vi "外观.vi"(0 "Data In":T9 caption="数据输入", 2 "Display State In":T2 caption="显示状态输入" {"配置信息"."间隔启动"."启动命令" items=["", "水样测试", "标样核查", "零点核查", "跨度核查", "空白测试", "平行样测试", "加标回收", "空白校准", "标样校准"]; "配置信息"."定点周期"."启动命令 24" items=["", "水样测试", "标样核查", "零点核查", "跨度核查", "空白测试", "平行样测试", "加标回收", "空白校准", "标样校准"]; "配置信息"."定点周期"."启动命令 23" items=["", "水样测试", "标样核查", "零点核查", "跨度核查", "空白测试", "平行样测试", "加标回收", "空白校准", "标样校准"]; "配置信息"."定点周期"."启动命令 22" items=["", "水样测试", "标样核查", "零点核查", "跨度核查", "空白测试", "平行样测试", "加标回收", "空白校准", "标样校准"]; "配置信息"."定点周期"."启动命令 21" items=["", "水样测试", "标样核查", "零点核查", "跨度核查", "空白测试", "平行样测试", "加标回收", "空白校准", "标样校准"]; "配置信息"."定点周期"."启动命令 20" items=["", "水样测试", "标样核查", "零点核查", "跨度核查", "空白测试", "平行样测试", "加标回收", "空白校准", "标样校准"]; "配置信息"."定点周期"."启动命令 19" items=["", "水样测试", "标样核查", "零点核查", "跨度核查", "空白测试", "平行样测试", "加标回收", "空白校准", "标样校准"]; "配置信息"."定点周期"."启动命令 18" items=["", "水样测试", "标样核查", "零点核查", "跨度核查", "空白测试", "平行样测试", "加标回收", "空白校准", "标样校准"]; "配置信息"."定点周期"."启动命令 17" items=["", "水样测试", "标样核查", "零点核查", "跨度核查", "空白测试", "平行样测试", "加标回收", "空白校准", "标样校准"]; "配置信息"."定点周期"."启动命令 16" items=["", "水样测试", "标样核查", "零点核查", "跨度核查", "空白测试", "平行样测试", "加标回收", "空白校准", "标样校准"]; "配置信息"."定点周期"."启动命令 15" items=["", "水样测试", "标样核查", "零点核查", "跨度核查", "空白测试", "平行样测试", "加标回收", "空白校准", "标样校准"]; "配置信息"."定点周期"."启动命令 14" items=["", "水样测试", "标样核查", "零点核查", "跨度核查", "空白测试", "平行样测试", "加标回收", "空白校准", "标样校准"]; "配置信息"."定点周期"."启动命令 13" items=["", "水样测试", "标样核查", "零点核查", "跨度核查", "空白测试", "平行样测试", "加标回收", "空白校准", "标样校准"]; "配置信息"."定点周期"."启动命令 12" items=["", "水样测试", "标样核查", "零点核查", "跨度核查", "空白测试", "平行样测试", "加标回收", "空白校准", "标样校准"]; "配置信息"."定点周期"."启动命令 11" items=["", "水样测试", "标样核查", "零点核查", "跨度核查", "空白测试", "平行样测试", "加标回收", "空白校准", "标样校准"]; "配置信息"."定点周期"."启动命令 10" items=["", "水样测试", "标样核查", "零点核查", "跨度核查", "空白测试", "平行样测试", "加标回收", "空白校准", "标样校准"]; "配置信息"."定点周期"."启动命令 9" items=["", "水样测试", "标样核查", "零点核查", "跨度核查", "空白测试", "平行样测试", "加标回收", "空白校准", "标样校准"]; "配置信息"."定点周期"."启动命令 8" items=["", "水样测试", "标样核查", "零点核查", "跨度核查", "空白测试", "平行样测试", "加标回收", "空白校准", "标样校准"]; "配置信息"."定点周期"."启动命令 7" items=["", "水样测试", "标样核查", "零点核查", "跨度核查", "空白测试", "平行样测试", "加标回收", "空白校准", "标样校准"]; "配置信息"."定点周期"."启动命令 6" items=["", "水样测试", "标样核查", "零点核查", "跨度核查", "空白测试", "平行样测试", "加标回收", "空白校准", "标样校准"]; "配置信息"."定点周期"."启动命令 5" items=["", "水样测试", "标样核查", "零点核查", "跨度核查", "空白测试", "平行样测试", "加标回收", "空白校准", "标样校准"]; "配置信息"."定点周期"."启动命令 4" items=["", "水样测试", "标样核查", "零点核查", "跨度核查", "空白测试", "平行样测试", "加标回收", "空白校准", "标样校准"]; "配置信息"."定点周期"."启动命令 3" items=["", "水样测试", "标样核查", "零点核查", "跨度核查", "空白测试", "平行样测试", "加标回收", "空白校准", "标样校准"]; "配置信息"."定点周期"."启动命令 2" items=["", "水样测试", "标样核查", "零点核查", "跨度核查", "空白测试", "平行样测试", "加标回收", "空白校准", "标样校准"]; "配置信息"."定点周期"."启动命令" items=["", "水样测试", "标样核查", "零点核查", "跨度核查", "空白测试", "平行样测试", "加标回收", "空白校准", "标样校准"]}, 3 "Container State":T8 caption="容器状态") -> (6 "Data Out":T9 caption="数据输出", 7 "Display State Out":T2 caption="显示状态输出" {"配置信息"."间隔启动"."启动命令" items=["", "水样测试", "标样核查", "零点核查", "跨度核查", "空白测试", "平行样测试", "加标回收", "空白校准", "标样校准"]; "配置信息"."定点周期"."启动命令 24" items=["", "水样测试", "标样核查", "零点核查", "跨度核查", "空白测试", "平行样测试", "加标回收", "空白校准", "标样校准"]; "配置信息"."定点周期"."启动命令 23" items=["", "水样测试", "标样核查", "零点核查", "跨度核查", "空白测试", "平行样测试", "加标回收", "空白校准", "标样校准"]; "配置信息"."定点周期"."启动命令 22" items=["", "水样测试", "标样核查", "零点核查", "跨度核查", "空白测试", "平行样测试", "加标回收", "空白校准", "标样校准"]; "配置信息"."定点周期"."启动命令 21" items=["", "水样测试", "标样核查", "零点核查", "跨度核查", "空白测试", "平行样测试", "加标回收", "空白校准", "标样校准"]; "配置信息"."定点周期"."启动命令 20" items=["", "水样测试", "标样核查", "零点核查", "跨度核查", "空白测试", "平行样测试", "加标回收", "空白校准", "标样校准"]; "配置信息"."定点周期"."启动命令 19" items=["", "水样测试", "标样核查", "零点核查", "跨度核查", "空白测试", "平行样测试", "加标回收", "空白校准", "标样校准"]; "配置信息"."定点周期"."启动命令 18" items=["", "水样测试", "标样核查", "零点核查", "跨度核查", "空白测试", "平行样测试", "加标回收", "空白校准", "标样校准"]; "配置信息"."定点周期"."启动命令 17" items=["", "水样测试", "标样核查", "零点核查", "跨度核查", "空白测试", "平行样测试", "加标回收", "空白校准", "标样校准"]; "配置信息"."定点周期"."启动命令 16" items=["", "水样测试", "标样核查", "零点核查", "跨度核查", "空白测试", "平行样测试", "加标回收", "空白校准", "标样校准"]; "配置信息"."定点周期"."启动命令 15" items=["", "水样测试", "标样核查", "零点核查", "跨度核查", "空白测试", "平行样测试", "加标回收", "空白校准", "标样校准"]; "配置信息"."定点周期"."启动命令 14" items=["", "水样测试", "标样核查", "零点核查", "跨度核查", "空白测试", "平行样测试", "加标回收", "空白校准", "标样校准"]; "配置信息"."定点周期"."启动命令 13" items=["", "水样测试", "标样核查", "零点核查", "跨度核查", "空白测试", "平行样测试", "加标回收", "空白校准", "标样校准"]; "配置信息"."定点周期"."启动命令 12" items=["", "水样测试", "标样核查", "零点核查", "跨度核查", "空白测试", "平行样测试", "加标回收", "空白校准", "标样校准"]; "配置信息"."定点周期"."启动命令 11" items=["", "水样测试", "标样核查", "零点核查", "跨度核查", "空白测试", "平行样测试", "加标回收", "空白校准", "标样校准"]; "配置信息"."定点周期"."启动命令 10" items=["", "水样测试", "标样核查", "零点核查", "跨度核查", "空白测试", "平行样测试", "加标回收", "空白校准", "标样校准"]; "配置信息"."定点周期"."启动命令 9" items=["", "水样测试", "标样核查", "零点核查", "跨度核查", "空白测试", "平行样测试", "加标回收", "空白校准", "标样校准"]; "配置信息"."定点周期"."启动命令 8" items=["", "水样测试", "标样核查", "零点核查", "跨度核查", "空白测试", "平行样测试", "加标回收", "空白校准", "标样校准"]; "配置信息"."定点周期"."启动命令 7" items=["", "水样测试", "标样核查", "零点核查", "跨度核查", "空白测试", "平行样测试", "加标回收", "空白校准", "标样校准"]; "配置信息"."定点周期"."启动命令 6" items=["", "水样测试", "标样核查", "零点核查", "跨度核查", "空白测试", "平行样测试", "加标回收", "空白校准", "标样校准"]; "配置信息"."定点周期"."启动命令 5" items=["", "水样测试", "标样核查", "零点核查", "跨度核查", "空白测试", "平行样测试", "加标回收", "空白校准", "标样校准"]; "配置信息"."定点周期"."启动命令 4" items=["", "水样测试", "标样核查", "零点核查", "跨度核查", "空白测试", "平行样测试", "加标回收", "空白校准", "标样校准"]; "配置信息"."定点周期"."启动命令 3" items=["", "水样测试", "标样核查", "零点核查", "跨度核查", "空白测试", "平行样测试", "加标回收", "空白校准", "标样校准"]; "配置信息"."定点周期"."启动命令 2" items=["", "水样测试", "标样核查", "零点核查", "跨度核查", "空白测试", "平行样测试", "加标回收", "空白校准", "标样校准"]; "配置信息"."定点周期"."启动命令" items=["", "水样测试", "标样核查", "零点核查", "跨度核查", "空白测试", "平行样测试", "加标回收", "空白校准", "标样校准"]}, 8 "Action":T1 caption="动作")   [LabVIEW 2016, in "定时设置.xctl"]
uses:
  <vilib>/_xctls/Container State.ctl
  <vilib>/_xctls/Action.ctl
  <vilib>/Utility/miscctls.llb/LVPositionTypeDef.ctl
  <vilib>/_xctls/XControlSupport.lvlib
  <vilib>/ptbypt/NI_PtbyPt.lvlib
panel:
  in  "周期设置":bool
  # "分钟"
  # "次"
  # "分钟"
  # "次"
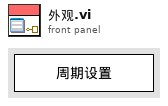
[diagram p1: front panel]
types:
  T1 = typedef "XControlSupport.lvlib/Action.ctl" = cluster{"Data Changed?":bool, "State Changed?":bool, "Action Name":string}
  T2 = typedef "定时设置.xctl/状态.ctl" = cluster{"配置信息":cluster{"周期模式":T3, "定点周期":T4, "间隔启动":T6, "测量参数":T7}, "仪器运行状态":bool, "启动次数":i32, "最近一次启动时间":timestamp, "最近一次结束时间":timestamp, "间隔计时":dbl, "测量参数名称":string[], "时间源":cluster{"时间源选择":enum16{"系统时间源", "仪器时间源"}, "外部时间源":timestamp}, "引用参数":string}
  T3 = typedef "定时设置.xctl/周期模式设置.ctl" = enum16{"不启用", "定点模式", "间隔模式"}
  T4 = typedef "定时设置.xctl/定点周期设置.ctl" = cluster{"启动命令":T5, "启动命令 2":T5, "启动命令 3":T5, "启动命令 4":T5, "启动命令 5":T5, "启动命令 6":T5, "启动命令 7":T5, "启动命令 8":T5, "启动命令 9":T5, "启动命令 10":T5, "启动命令 11":T5, "启动命令 12":T5, "启动命令 13":T5, "启动命令 14":T5, "启动命令 15":T5, "启动命令 16":T5, "启动命令 17":T5, "启动命令 18":T5, "启动命令 19":T5, "启动命令 20":T5, "启动命令 21":T5, "启动命令 22":T5, "启动命令 23":T5, "启动命令 24":T5}
  T5 = typedef "定时设置.xctl/启动命令选择.ctl" = u16
  T6 = typedef "定时设置.xctl/间隔启动设置.ctl" = cluster{"启动命令":T5, "启动间隔":dbl, "启动次数":i32}
  T7 = typedef "定时设置.xctl/测量参数.ctl" = u16
  T8 = typedef "XControlSupport.lvlib/Container State.ctl" = cluster{"Indicator?":bool, "Run Mode?":bool, " Refnum":refnum<vi>}
  T9 = typedef "定时设置.xctl/数据.ctl" = cluster{"启动":bool, "控制命令":T10, "测量参数":T7}
  T10 = typedef "定时设置.xctl/国标控制命令.ctl" = enum16{"启动测量", "标样核查", "零点核查", "跨度核查", "空白测试", "平行样测试", "加标回收", "空白校准", "标样校准", "初始化（清洗）", "停止测试", "仪器重启", "校时", "模式设置", "测量间隔设置"}
  T11 = typedef "LVPositionTypeDef.ctl" = cluster{"Left":i32, "Top":i32}
  T12 = cluster{"周期模式":T3, "定点周期":T4, "间隔设置":cluster{"启动命令":T5, "启动间隔":dbl, "启动次数":i32}, "测量参数":T7}
  T13 = cluster{"周期模式":T3, "定点周期":T4, "间隔启动":T6, "测量参数":T7}
  T14 = cluster{"时间源选择":enum16{"系统时间源", "仪器时间源"}, "外部时间源":timestamp}
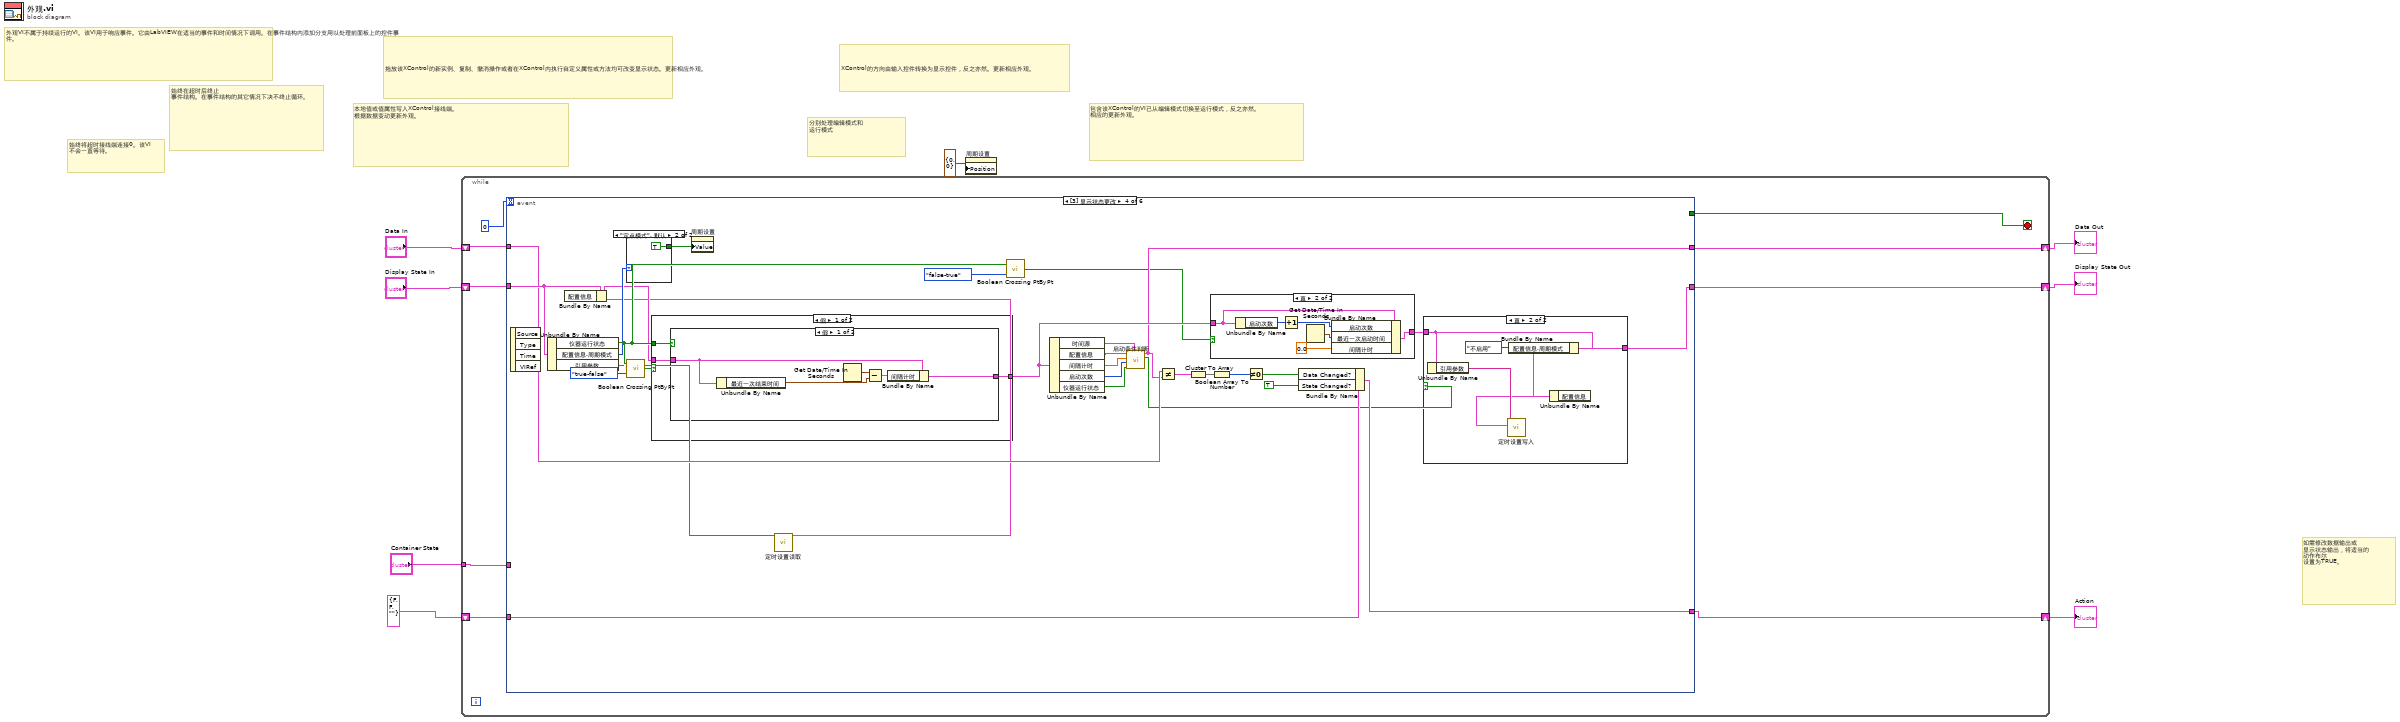
[diagram p0: block diagram]
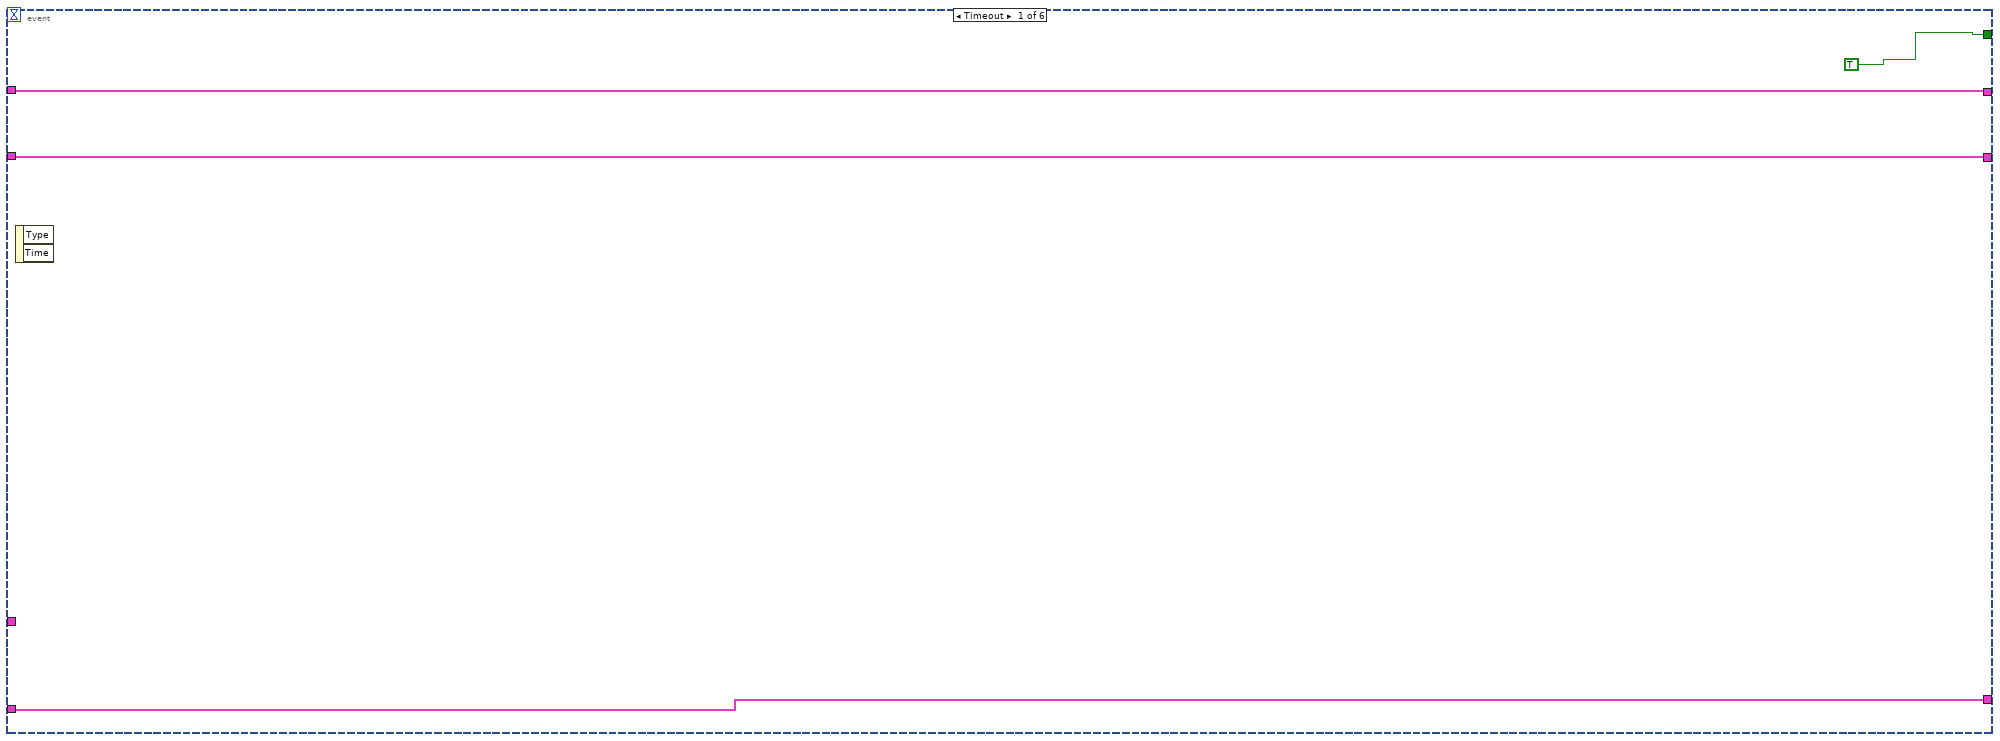
[diagram p2: hidden frame]
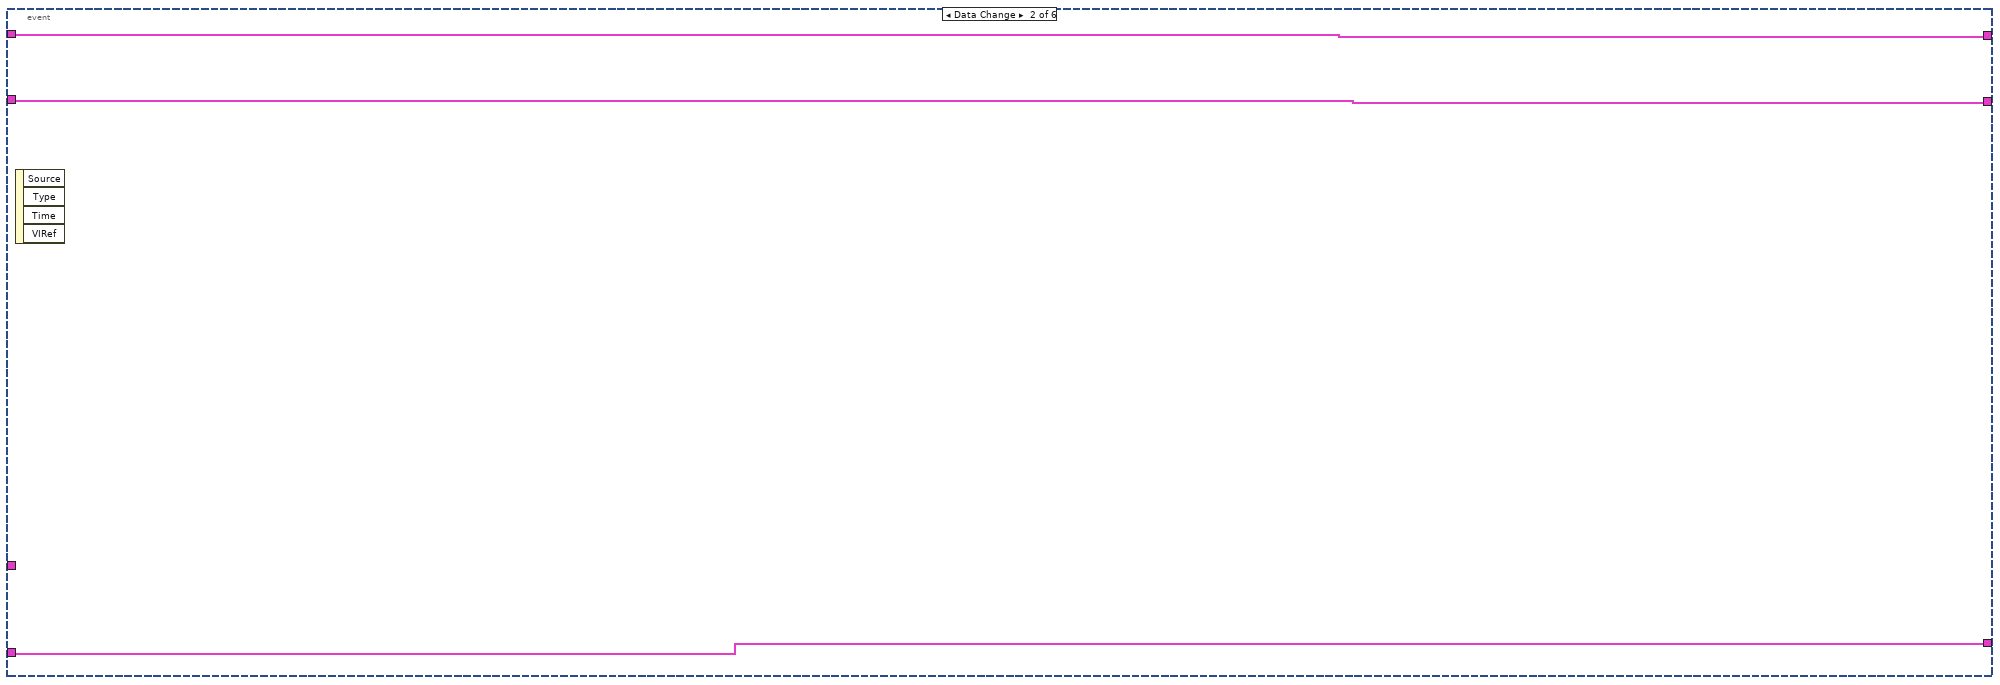
[diagram p3: hidden frame]
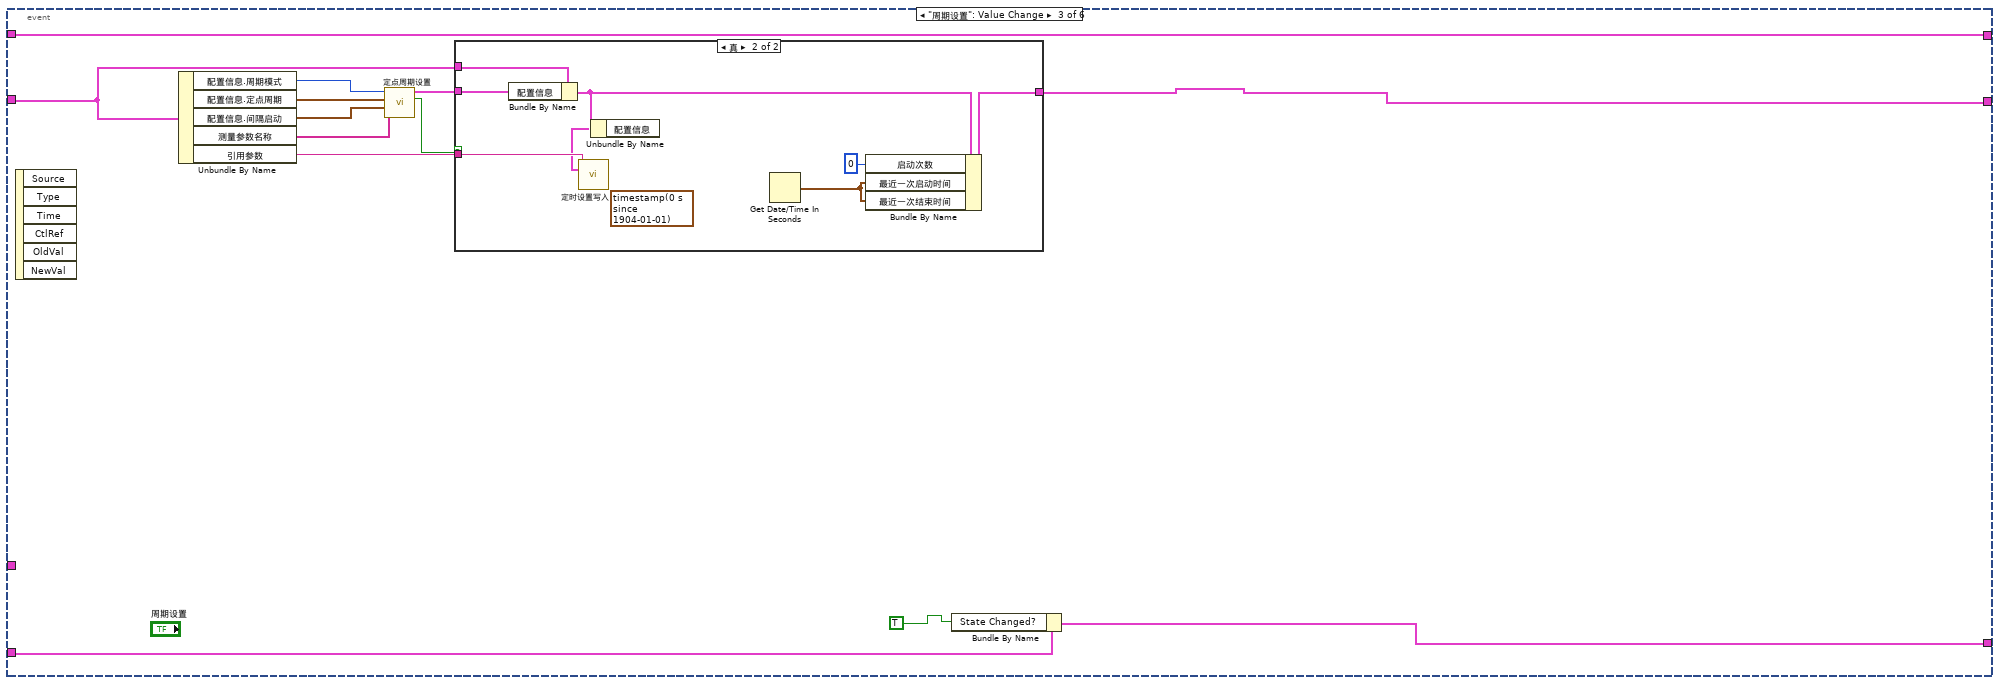
[diagram p4: hidden frame]
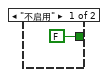
[diagram p7: hidden frame]
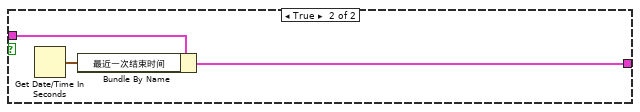
[diagram p9: hidden frame]
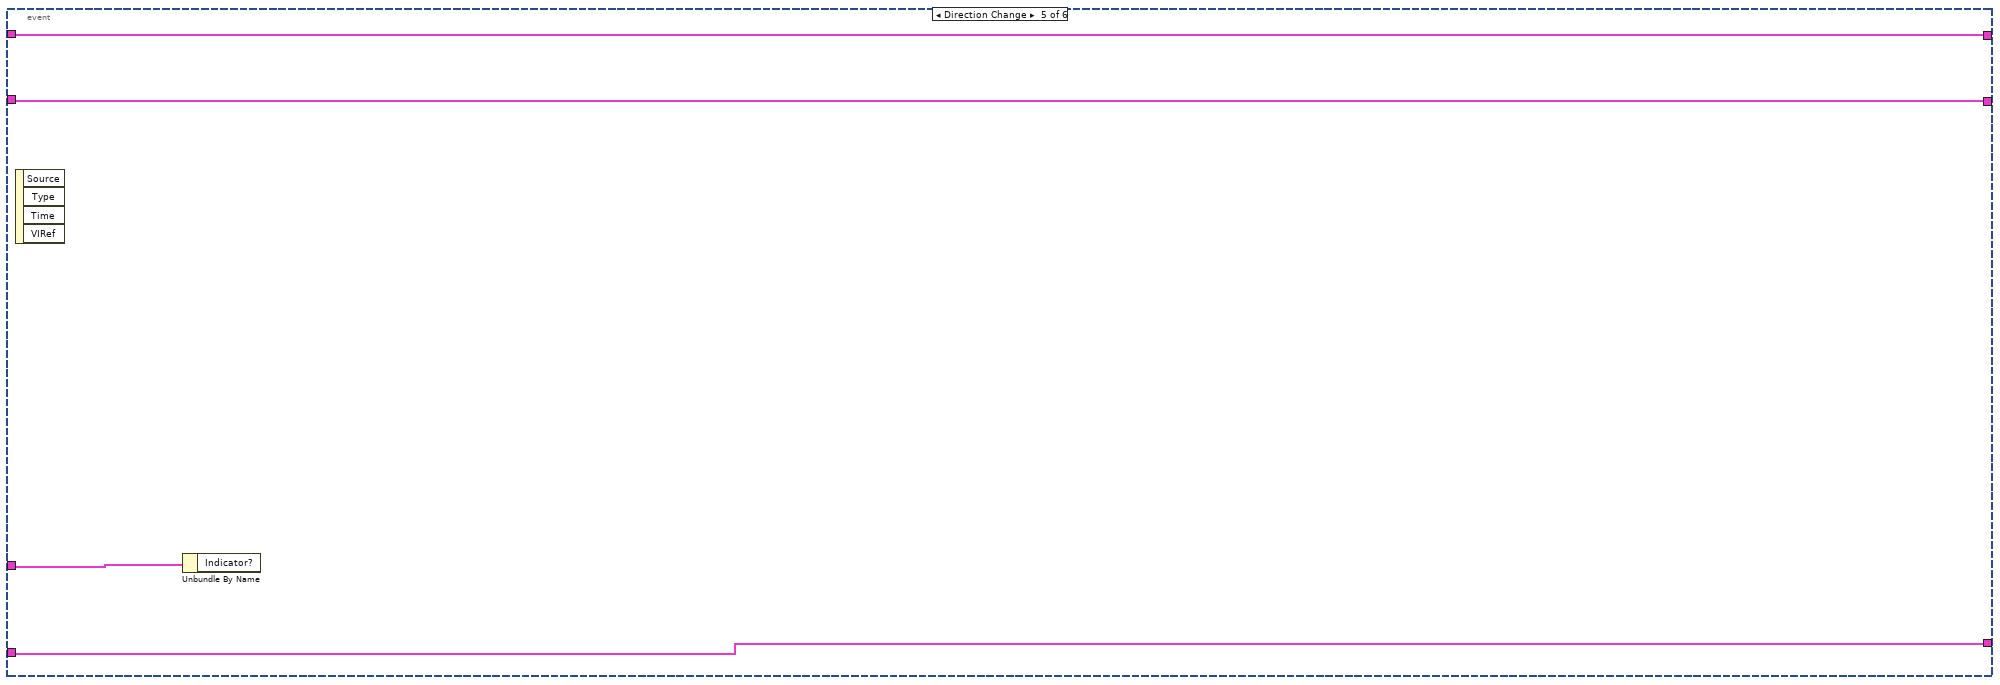
[diagram p11: hidden frame]
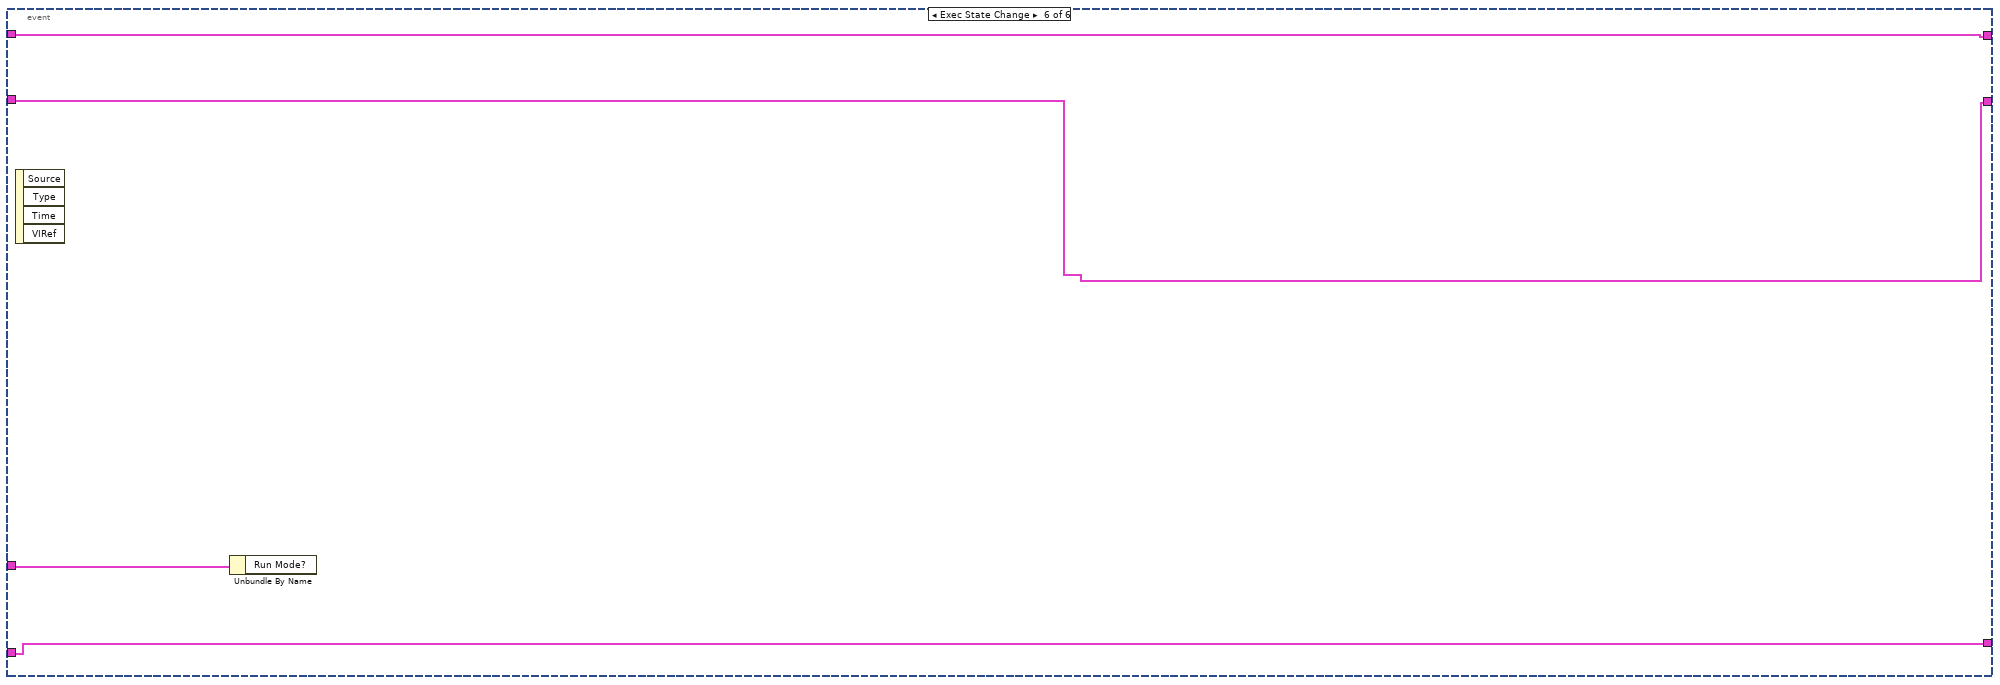
[diagram p12: hidden frame]
diagram:
  # "分别处理编辑模式和\n运行模式"
  # "包含该XControl的VI已从编辑模式切换至运行模式，反之亦然。\n相应的更新外观。"
  # "XControl的方向由输入控件转换为显示控件，反之亦然。更新相应外观。"
  # "始终将超时接线端连接0。该VI\n不会一直等待。"
  # "拖放该XControl的新实例、复制、撤消操作或者在XControl内执行自定义属性或方法均可改变显示状态。更新相应外观。"
  # "本地值或值属性写入XControl接线端。\n根据数据变动更新外观。"
  # "始终在超时后终止\n事件结构。在事件结构的其它情况下决不终止循环。"
  # "外观VI不属于持续运行的VI。该VI用于响应事件。它由LabVIEW在适当的事件和时间情况下调用。在事件结构内添加分支用以处理前面板上的控件事件。"
  # "如需修改数据输出或\n显示状态输出，将适当的\n动作布尔\n设置为TRUE。"
  n1 = while {
    shift-right: [w16] -> w5
    shift-left: "Display State In" -> [w17]
    tunnel: "Container State" -> [w13]
    shift-right: [w11] -> w8
    shift-left: "Data In" -> [w12]
    shift-right: [w9] -> w3
    shift-left: T1 {"Data Changed?"=FALSE, "State Changed?"=FALSE, "Action Name"=""} ("Action") -> [w10]
    stop <- w15 stop-if-true
    n2 = event shown="[3] 显示状态更改" {
      selector: _ -> [_ _ _ _ _ _]
      dyn-events: _ -> [_ _ _ _ _ _]
      timeout: 0 -> [_ _ _ _ _ _]
      tunnel: w17 -> [w19 w23 w34 w70 w105 w107]
      tunnel: [w19 w23 w27 w54 w105 w107] -> w16
      tunnel: [TRUE _ _ _ _ _] -> w15
      tunnel: w13 -> [_ _ _ _ w106 w110]
      tunnel: w12 -> [w18 w24 w35 w62 w104 w108]
      tunnel: [w18 w24 w35 w61 w104 w108] -> w11
      tunnel: [w20 w22 w32 w73 w103 w109] -> w9
      tunnel: w10 -> [w20 w22 w33 w74 w103 w109]
      event Timeout {
        n3 = event-data() -> ()  [unwired: 1 in, 2 out]
      }
      event Data Change {
        n4 = event-data() -> ()  [unwired: 1 in, 4 out]
      }
      event "周期设置": Value Change {
        n5 = event-data() -> ()  [unwired: 1 in, 6 out]
        n6 = Unbundle By Name(w34) -> ("配置信息.周期模式"=w29:T3, "配置信息.定点周期"=w36:T4, "配置信息.间隔启动"=w37:T6, "测量参数名称"=w26:string[], "引用参数"=w25:string)
        n7 = call "定点周期设置.vi"("测量参数字符串[]"=w26, "间隔启动"=w37, "定点周期"=w36, "周期模式"=w29) -> ("保存输出"=w28:bool, "周期设置输出"=w30:T12)  [unwired: 6 in]
        n8 = case shown="真" w28 {
          tunnel: w34 -> [w38 w46]
          tunnel: [w38 w45] -> w27
          tunnel: w30 -> [_ w42]
          tunnel: w25 -> [_ w43]
          frame False {
          }
          frame True {
            (unwired) timestamp(0 s since 1904-01-01) ("最近一次启动时间")
            n9 = Bundle By Name(cluster=w46, "配置信息"=w42) -> (w41:T2)
            n10 = Unbundle By Name(w41) -> ("配置信息"=w40:T13)
            n11 = call "定时设置写入.vi"("INI Fomatted Cluster"=w40, "测试参数"=w43) -> ()  [unwired: 10 in]
            n12 = Get Date/Time In Seconds() -> (seconds since 1Jan1904=w39:timestamp)
            n13 = Bundle By Name(cluster=w41, "启动次数"=0, "最近一次启动时间"=w39, "最近一次结束时间"=w39) -> (w45:T2)
          }
        }
        n14 = Bundle By Name(cluster=w33, "State Changed?"=TRUE) -> (w32:T1)
      }
      event Display State Change {
        n15 = event-data() -> ()  [unwired: 1 in, 4 out]
        n16 = Unbundle By Name(w70) -> ("仪器运行状态"=w52:bool, "配置信息.周期模式"=w64:T3, "引用参数"=w49:string)
        n17 = case shown="\"定点模式\", 默认" w64 {
          tunnel: [FALSE TRUE] -> w63
          frame "不启用" {
          }
          frame "定点模式", Default {
          }
        }
        n18 = call <vilib>:"Boolean Crossing PtByPt.vi"("direction"=enum16{"either", "false-true", "true-false"}."true-false", "input"=w52) -> ("crossing"=w71:bool)  [unwired: 1 in]
        n19 = property on="周期设置" class="Bool (严格)"("Value"=w63) -> ()  [unwired: 2 in, 2 out]
        n20 = call "定时设置读取.vi"("引用参数"=w49) -> ("周期设置输出"=w47:T13)  [unwired: 10 in]
        n21 = Bundle By Name(cluster=w70, "配置信息"=w47) -> (w48:T2)
        n22 = case shown="假" w71 {
          tunnel: w48 -> [w86 w95]
          tunnel: [w85 w94] -> w69
          tunnel: w52 -> [w84 _]
          frame False {
            n23 = case shown="假" w84 {
              tunnel: w86 -> [w90 w92]
              tunnel: [w88 w92] -> w85
              frame False {
                n24 = Unbundle By Name(w90) -> ("最近一次结束时间"=w87:timestamp)
                n25 = Get Date/Time In Seconds() -> (seconds since 1Jan1904=w91:timestamp)
                n26 = Subtract(x=w91, y=w87) -> (x-y=w89:dbl)
                n27 = Bundle By Name(cluster=w90, "间隔计时"=w89) -> (w88:T2)
              }
              frame True {
              }
            }
          }
          frame True {
            n28 = Get Date/Time In Seconds() -> (seconds since 1Jan1904=w93:timestamp)
            n29 = Bundle By Name(cluster=w95, "最近一次结束时间"=w93) -> (w94:T2)
          }
        }
        n30 = call <vilib>:"Boolean Crossing PtByPt.vi"("direction"=enum16{"either", "false-true", "true-false"}."false-true", "input"=w52) -> ("crossing"=w51:bool)  [unwired: 1 in]
        n31 = Unbundle By Name(w69) -> ("时间源"=w50:T14, "配置信息"=w68:T13, "间隔计时"=w67:dbl, "启动次数"=w66:i32, "仪器运行状态"=w65:bool)
        n32 = call "启动条件判断.vi"("时间源"=w50, "仪器状态"=w65, "启动次数"=w66, "间隔计时"=w67, "周期设置输出"=w68) -> ("重新配置"=w55:bool, "Data"=w61:T9)  [unwired: 5 in]
        n33 = Not Equal?(x=w62, y=w61) -> (x != y?=w60:cluster{"启动":bool, "控制命令":bool, "测量参数":bool})
        n34 = Cluster To Array(cluster=w60) -> (array=w59:bool[])
        n35 = case shown="真" w51 {
          tunnel: w69 -> [w96 w100]
          tunnel: [w96 w102] -> w56
          frame False {
          }
          frame True {
            n36 = Unbundle By Name(w100) -> ("启动次数"=w99:i32)
            n37 = Increment(x=w99) -> (x+1=w98:i32)
            n38 = Get Date/Time In Seconds() -> (seconds since 1Jan1904=w101:timestamp)
            n39 = Bundle By Name(cluster=w100, "启动次数"=w98, "最近一次启动时间"=w101, "间隔计时"=0.0) -> (w102:T2)
          }
        }
        n40 = Boolean Array To Number(Boolean array=w59) -> (number=w58:u32)
        n41 = Not Equal To 0?(x=w58) -> (x != 0?=w57:bool)
        n42 = Bundle By Name(cluster=w74, "Data Changed?"=w57, "State Changed?"=TRUE) -> (w73:T1)
        n43 = case shown="真" w55 {
          tunnel: w56 -> [w76 w79]
          tunnel: [w76 w80] -> w54
          frame False {
          }
          frame True {
            n44 = Unbundle By Name(w79) -> ("引用参数"=w78:string)
            n45 = Bundle By Name(cluster=w79, "配置信息.周期模式"=周期模式设置."不启用") -> (w80:T2)
            n46 = Unbundle By Name(w80) -> ("配置信息"=w77:T13)
            n47 = call "定时设置写入.vi"("INI Fomatted Cluster"=w77, "测试参数"=w78) -> ()  [unwired: 10 in]
          }
        }
      }
      event Direction Change {
        n48 = event-data() -> ()  [unwired: 1 in, 4 out]
        n49 = Unbundle By Name(w106) -> ()  [unwired: 1 out]
      }
      event Exec State Change {
        n50 = event-data() -> ()  [unwired: 1 in, 4 out]
        n51 = Unbundle By Name(w110) -> ()  [unwired: 1 out]
      }
    }
  }
  "Display State Out" <- w5
  "Data Out" <- w8
  "Action" <- w3
  n52 = property on="周期设置" class="Bool (严格)"("Position"=T11 {"Left"=0, "Top"=0} ("位置")) -> ()  [unwired: 2 in, 2 out]
